vi "Write commandFactory.vi"(10 "ICommandFactory.lvclass":refnum<class "ICommandFactory.lvclass">, 11 "CommandConstruction in":refnum<class "CommandConstruction.lvclass">) -> (3 "CommandConstruction out":refnum<class "CommandConstruction.lvclass">)   [LabVIEW 2016, in "CommandConstruction.lvclass"]
uses:
  CommandConstruction.lvclass
  ICommandFactory/ICommandFactory.lvclass
  CommandConstruction.lvclass/CommandConstruction.ctl
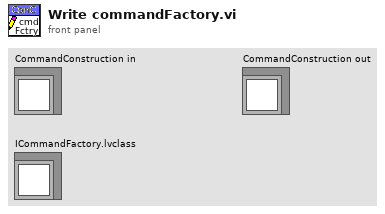
[diagram p1: front panel]
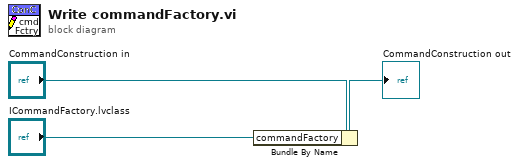
[diagram p0: block diagram]
diagram:
  n1 = Bundle By Name(cluster="CommandConstruction in", "commandFactory"="ICommandFactory.lvclass") -> (→"CommandConstruction out":refnum<class "CommandConstruction.lvclass">)
